vi "GetAcquiredDataSD.vi"(0 "size":u32, 1 "error in (no error)":errorcluster) -> (2 "array":i32[](array[numeric]), 3 "DLL error code":u32, 4 "error out":errorcluster)   [LabVIEW 2015]
doc: "This function will return the data from the last acquisition. The data are returned as long integers (32-bit signed integers).\n\n<B>Parameters</B>:\nsize - total number of pixels.\narray - data storage.\n\n<B>Error codes:</B>\nDRV_SUCCESS - Data copied.\nDRV_NOT_INITIALIZED - System not initialized.\nDRV_ACQUIRING - Acquisition in progress.\nDRV_ERROR_ACK - Unable to communicate with card.\nDRV_P1INVALID - Invalid pointer (i.e. NULL).\nDRV_P2INVALID - Array size is too small."
uses:
  DLL/atmcd32d.dll
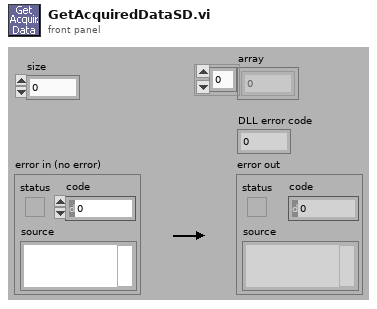
[diagram p1: front panel]
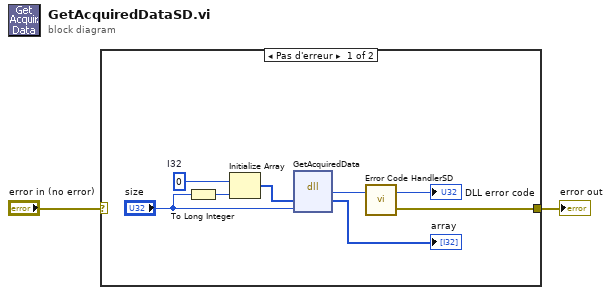
[diagram p0: block diagram]
diagram:
  n1 = case shown="Pas d'erreur" "error in (no error)" {
    selector: "error in (no error)" -> [_ w11]
    tunnel: [w9 w11] -> w1
    frame No Error {
      w5 = 0  # I32
      n2 = To Long Integer(number="size") -> (32bit integer=w3:i32)
      n3 = Initialize Array "Initialize Array"(w5, w3) -> (w4:i32[])
      n4 = dll-call lib="G:/SD/TRANCON/DLL/Atmcd32d.dll" fn="GetAcquiredData"("array"=w4, "size"="size") -> (w10:u32, "array"=→"array":i32[])  [unwired: 4 in, 2 out]
      n5 = call "Error Code HandlerSD.vi"("DLL error code"=w10) -> ("error out"=w9:errorcluster, "dup DLL error code"=→"DLL error code":u32)  [unwired: 1 in]
    }
    frame Error {
    }
  }
  "error out" <- w1
